vi "UHR-Fleezers Control (host) - 16.2.2v2.vi"() -> ()   [LabVIEW 2014] (continued)
                            n638 = Greater Or Equal?(x=w963, y="Dwell Duration (s)") -> (x >= y?=w970:bool)
                            n639 = local read "Dip for Protein"() -> (w967:bool)
                            n640 = Not(x=w967) -> (.not. x?=w966:bool)
                            n641 = Compound Arithmetic op=OR(w970, "Cancel dwell", w966) -> (w969:bool)
                            n642 = node-c288() -> ()  [unwired: 1 in, 1 out]
                            n643 = Select(t=FALSE, s="Pause dwell", f=w969) -> (s? t:f=w972:bool)
                            n644 = Or(x=w972, y=w964) -> (x .or. y?=w965:bool)
                            "Dwell Time (s)" <- w963
                          }
                          n645 = node-c288(w961) -> ()  [unwired: 1 out]
                        }
                      }
                    }
                  }
                }
                frame #4 {
                  n646 = local read "Dip for Protein"() -> (w982:bool)
                  n647 = local read "Dump Beads"() -> (w979:bool)
                  n648 = local write "Cancel dwell"(FALSE ("Cancel dwell")) -> ()
                  n649 = Not(x=w982) -> (.not. x?=w983:bool)
                  n650 = Not(x="Cont. Repeat Dipping?") -> (.not. x?=w985:bool)
                  n651 = Compound Arithmetic op=OR(w983, w985, w979) -> (w981:bool)
                }
              }
            }
          }
        }
      }
      event "Profile": Value Change {
        n652 = event-data() -> ()  [unwired: 1 in, 5 out]
        n653 = flat-sequence {
          tunnel: w994 -> [w997]
          tunnel: w993 -> [w1005]
          tunnel: [w999] -> w992
          tunnel: [w998] -> w991
          tunnel: [w996] -> w989
          tunnel: [w995] -> w986
          tunnel: w992 -> [w1012]
          tunnel: w991 -> [w1011]
          tunnel: [w1009] -> w990
          tunnel: w989 -> [w1010]
          tunnel: [w1008] -> w988
          tunnel: [w1007] -> w987
          tunnel: w986 -> [w1007]
          tunnel: w990 -> [w1016]
          tunnel: w988 -> [w1015]
          tunnel: w987 -> [w1014]
          frame #0 {
            n654 = call "Read Stage Position.vi"("error in"=w1005, "VISA resource name in"=w997) -> ("Current Position"=w995:cluster{dbl, dbl, dbl}, "error out"=w998:errorcluster, "VISA resource name out"=w996:refnum<visa-resource-name>)  [unwired: 1 out]
            "Current Position" <- w995
            n655 = local write "Stage Control Serial Error"(w998) -> ()
            n656 = Unbundle(w995) -> (w1002:dbl, w1004:dbl, w1000:dbl)
            n657 = Add(x=w1004, y="Y change (mm)") -> (x+y=w1001:dbl)
            n658 = Bundle(w1002, w1001, w1000) -> (w999:cluster{dbl, dbl, dbl})  [unwired: 1 in]
          }
          frame #1 {
            # "move to new position and start saving"
            n659 = local write "Stage Moving"(TRUE ("Stage Moving")) -> ()
            n660 = local write "Start Saving"(TRUE ("Start Saving")) -> ()
            n661 = call "Set Stage Position.vi"("Position"=w1012, "error in"=w1011, "VISA resource name in"=w1010) -> ("error out"=w1008:errorcluster, "VISA resource name out"=w1009:refnum<visa-resource-name>)  [unwired: 1 out]
          }
          frame #2 {
            # "go back to start"
            n662 = call "Set Stage Position.vi"("Position"=w1014, "error in"=w1015, "VISA resource name in"=w1016) -> ()  [unwired: 3 out]
          }
          frame #3 {
            # "stop saving"
            n663 = local write "Stop Saving"(TRUE ("Stop Saving")) -> ()
            n664 = local write "Stage Moving"(FALSE ("Stage Moving")) -> ()
          }
        }
      }
      event "Move to Position 1", "Move to Position 2", "Move to Position 3", "Move to Position 4", "Move to Position 5", "Lower Ch. Cap.", "Move to Position 6": Value Change {
        n665 = event-data() -> ()  [unwired: 1 in, 5 out]
        n666 = Or(x="Move to Position 5", y="Lower Ch. Cap.") -> (x .or. y?=w1023:bool)
        n667 = Build Array("Move to Position 1", "Move to Position 2", "Move to Position 3", "Move to Position 4", w1023, "Move to Position 6") -> (w1026:bool[])
        n668 = Boolean Array To Number(Boolean array=w1026) -> (number=w1025:u32)
        n669 = Logarithm Base 2(1:w1025) -> (0:w1024:dbl)
        n670 = flat-sequence {
          tunnel: w1024 -> [w1035]
          tunnel: w1021 -> [w1033]
          tunnel: w1020 -> [w1032]
          frame #0 {
            n671 = local read "Saved Stage Positions"() -> (w1043:dbl[][])
            n672 = Array Subset(array=w1043, index (row)=w1035, length (row)=1 ("length"), index (col)=1 ("index"), length (col)=3 ("length")) -> (w1040:dbl[][])
            n673 = Reshape Array(w1040, 3 ("dimension size")) -> (w1038:dbl[])
            n674 = Array To Cluster(array=w1038) -> (cluster=w1037:cluster{"[0]":dbl, "[1]":dbl, "[2]":dbl})
            n675 = call "Set Stage Position.vi"("Position"=w1037, "error in"=w1032, "VISA resource name in"=w1033) -> ("error out"=w1036:errorcluster)  [unwired: 2 out]
            n676 = local write "Stage Moving"(TRUE ("Stage Moving")) -> ()
            n677 = local write "Stage Control Serial Error"(w1036) -> ()
          }
          frame #1 {
            n678 = local write "Stage Moving"(FALSE ("Stage Moving")) -> ()
            n679 = call <vilib>:"Beep.vi"() -> ()  [unwired: 3 in, 9 out]
          }
        }
      }
      event "Got ADig bead": Value Change {
        n680 = event-data() -> ()  [unwired: 1 in, 5 out]
        n681 = flat-sequence {
          frame #0 {
            n682 = local read "Cap 1 Samp Flow ON"() -> (w1047:bool)
            n683 = case shown="True" w1047 {
              frame False {
              }
              frame True {
                n684 = property on="Sample Channel\nFlow" class="Bool (strict)"("Val(Sgnl)"=TRUE ("Value (Signaling)")) -> ()  [unwired: 2 in, 2 out]
              }
            }
          }
          frame #1 {
            n685 = property on="Inject Pump 3" class="Bool (strict)"("Val(Sgnl)"=FALSE ("Value (Signaling)")) -> ()  [unwired: 2 in, 2 out]
          }
          frame #2 {
            n686 = property on="Move Cap. 1 (DNA Bottom)" class="Bool (strict)"("Val(Sgnl)"=TRUE ("Value (Signaling)")) -> ()  [unwired: 2 in, 2 out]
          }
        }
      }
      event "Force FB Data\nScript": Value Change {
        n687 = event-data() -> ()  [unwired: 1 in, 5 out]
        n688 = flat-sequence {
          tunnel: w1056 -> [w1060]
          tunnel: w1057 -> [w1061]
          tunnel: [w1061] -> w1052
          tunnel: [w1060] -> w1051
          tunnel: w1052 -> [w1064]
          tunnel: w1051 -> [w1063]
          tunnel: ["Trap Trig Fl."] -> w1053
          tunnel: [w1089] -> w1054
          tunnel: w1053 -> [w1089]
          tunnel: [w1093] -> w1055
          tunnel: w1054 -> [w1093]
          tunnel: w1055 -> [w1095]
          frame #0 {
            n689 = property on="Trap Delta (MHz)" class="DigNum (strict)"("Val(Sgnl)"="Trap Delta Before Moving") -> ()  [unwired: 2 in, 2 out]
          }
          frame #1 {
            n690 = local read "Saved Stage Positions"() -> (w1066:dbl[][])
            n691 = property on="Trap Pos. FB Offset Factor" class="DigNum (strict)"("Val(Sgnl)"=i64 0 ("Value (Signaling)")) -> ()  [unwired: 2 in, 2 out]
            n692 = local write "FB Trap Pos Offset"(0.0 ("FB Trap Pos Offset")) -> ()
            n693 = local write "Stage Moving"(TRUE ("Stage Moving")) -> ()
            n694 = call "move to saved stage position.vi"("error in"=w1063, "Stage VISA resource name in"=w1064, "Position"="Stage Position To Establish FB", "Saved Stage Positions"=w1066) -> ("error out"=w1062:errorcluster)  [unwired: 1 out]
            n695 = local write "Stage Control Serial Error"(w1062) -> ()
          }
          frame #2 {
            n696 = call <vilib>:"Beep.vi"() -> ()  [unwired: 3 in, 9 out]
            n697 = Multiply(x="Wait (s)", y=u32 1000 ("milliseconds to wait")) -> (x*y=w1073:u32)
            n698 = property on="Trap Delta (MHz)" class="DigNum (strict)"("Val(Sgnl)"="Starting \nTrap Delta (MHz)") -> ()  [unwired: 2 in, 2 out]
            n699 = local write "Stage Moving"(FALSE ("Stage Moving")) -> ()
            n700 = Wait (ms)(milliseconds to wait=w1073) -> ()  [unwired: 1 out]
            n701 = property on="Tab Control 2" class="TabCtl (strict)"("Val(Sgnl)"=T8."Feedback on Trap Position" ("Value (Signaling)")) -> ()  [unwired: 2 in, 2 out]
            n702 = property on="Tab Control" class="TabCtl (strict)"("Val(Sgnl)"=T32."Trap Control (RF)" ("Value (Signaling)")) -> ()  [unwired: 2 in, 2 out]
          }
          frame #3 {
            n703 = property on="Set Reading to\nSetpoint" class="Bool (strict)"("Val(Sgnl)"=TRUE ("Value (Signaling)")) -> ()  [unwired: 2 in, 2 out]
            n704 = Wait (ms)(milliseconds to wait=u32 500) -> ()  [unwired: 1 out]
          }
          frame #4 {
            n705 = property on="Trap Pos. FB ON" class="Bool (strict)"("Val(Sgnl)"=TRUE ("Value (Signaling)")) -> ()  [unwired: 2 in, 2 out]
            n706 = Wait (ms)(milliseconds to wait=u32 250) -> ()  [unwired: 1 out]
          }
          frame #5 {
            n707 = case shown="False" "Trap Trig Fl." {
              frame False {
                n708 = case shown="True" "Green ON after FB ON?" {
                  selector: "Green ON after FB ON?" -> [_ w1088]
                  frame False {
                  }
                  frame True {
                    n709 = property on="Green Laser ON" class="Bool (strict)"("Val(Sgnl)"=w1088) -> ()  [unwired: 2 in, 2 out]
                  }
                }
              }
              frame True {
              }
            }
            n710 = case shown="True" "Remove Action Offset" {
              tunnel: TRUE ("Value (Signaling)") -> [w1085 w1086]
              frame False {
                n711 = property on="Remove Unwinding Offset" class="Bool (strict)"("Val(Sgnl)"=w1085) -> ()  [unwired: 2 in, 2 out]
              }
              frame True {
                n712 = property on="Remove Action Offset" class="Bool (strict)"("Val(Sgnl)"=w1086) -> ()  [unwired: 2 in, 2 out]
              }
            }
            n713 = Wait (ms)(milliseconds to wait=u32 250) -> ()  [unwired: 1 out]
          }
          frame #6 {
            n714 = property on="Start Saving" class="Bool (strict)"("Val(Sgnl)"=TRUE ("Value (Signaling)")) -> ()  [unwired: 2 in, 2 out]
            n715 = Wait (ms)(milliseconds to wait=u32 5000) -> ()  [unwired: 1 out]
          }
          frame #7 {
            w1092 = TRUE ("Value (Signaling)")
            n716 = property on="Rem fb disp offset" class="Bool (strict)"("Val(Sgnl)"=w1092) -> ()  [unwired: 2 in, 2 out]
            n717 = property on="Remove Offset" class="Bool (strict)"("Val(Sgnl)"=w1092) -> ()  [unwired: 2 in, 2 out]
            n718 = Wait (ms)(milliseconds to wait=u32 100) -> ()  [unwired: 1 out]
          }
          frame #8 {
            n719 = case shown="True" w1095 {
              frame False {
              }
              frame True {
                n720 = local write "Trap Trig. Fl."(TRUE ("Value (Signaling)")) -> ()
              }
            }
          }
          frame #9 {
            n721 = case shown="True" "Start dipping after?" {
              frame False {
              }
              frame True {
                n722 = flat-sequence {
                  frame #0 {
                    n723 = Multiply(x="Delay before dipping (s)", y=1000.0) -> (x*y=w1099:dbl)
                    n724 = Wait (ms)(milliseconds to wait=w1099) -> ()  [unwired: 1 out]
                  }
                  frame #1 {
                    n725 = property on="Dip for Protein" class="Bool (strict)"("Val(Sgnl)"=TRUE ("Value (Signaling)")) -> ()  [unwired: 2 in, 2 out]
                    n726 = local write "Scripts"(T33."Dipping" ("Scripts")) -> ()
                  }
                }
              }
            }
          }
        }
      }
      event "Start lifetime measurements": Value Change {
        n727 = event-data() -> ()  [unwired: 1 in, 5 out]
        n728 = local write "Start lifetime measurements"(FALSE ("Start lifetime measurements")) -> ()
        n729 = flat-sequence {
          tunnel: w1104 -> [w1107]
          tunnel: [w1107] -> w1103
          tunnel: w1103 -> [w1114]
          frame #0 {
            # "This will:\n1) stop reading trap pos fifo\n2) start sending zeros to trap position host data\nWait a second because may be in the middle of\nwaiting for FIFO data."
            n730 = local write "Trap positions to FIFO"(FALSE ("Trap positions to FIFO")) -> ()
            n731 = Wait (ms)(milliseconds to wait=u32 1000) -> ()  [unwired: 1 out]
          }
          frame #1 {
            w1113 = FALSE ("Trap Pos to FIFO")
            # "Send lifetimes to FIFO"
            # "Stop and restart FIFO to clear"
            # "On FPGA, stop sending trap\nposition data to FIFO and make\nsure lifetimes aren't sent to FIFO\neither"
            n732 = xnode "Read/Write Control"("FPGA VI Reference In"=w1114, "Trap Pos to FIFO"=w1113, "Lifetime to FIFO"=w1113, "lifetime events in fifo"=u16 0) -> ("FPGA VI Reference Out"=w1115:T25)  [unwired: 1 in, 1 out]
            n733 = xnode "Invoke Method"("FPGA VI Reference In"=w1115) -> ("FPGA VI Reference Out"=w1112:T25)  [unwired: 1 in, 1 out]
            n734 = xnode "Invoke Method"("FPGA VI Reference In"=w1112) -> ("FPGA VI Reference Out"=w1111:T25)  [unwired: 1 in, 1 out]
            n735 = xnode "Read/Write Control"("FPGA VI Reference In"=w1111, "Lifetime to FIFO"=TRUE) -> ()  [unwired: 1 in, 2 out]
          }
          frame #2 {
            "Measuring lifetimes" <- TRUE ("Measuring lifetimes")
          }
        }
      }
      event "Stop lifetime measurements": Value Change {
        n736 = event-data() -> ()  [unwired: 1 in, 5 out]
        n737 = local write "Stop lifetime measurements"(FALSE ("Stop lifetime measurements")) -> ()
        n738 = flat-sequence {
          tunnel: w1117 -> [w1126]
          frame #0 {
            n739 = local write "Measuring lifetimes"(FALSE ("Measuring lifetimes")) -> ()
          }
          frame #1 {
            # "clear fifo count"
            # "Start sending trap position\ndata to FIFO"
            # "Stop sending lifetime data\nto FIFO"
            n740 = xnode "Read/Write Control"("FPGA VI Reference In"=w1126, "Lifetime to FIFO"=FALSE ("Trap Pos to FIFO")) -> ("FPGA VI Reference Out"=w1125:T25)  [unwired: 1 in, 1 out]
            n741 = xnode "Read/Write Control"("FPGA VI Reference In"=w1125, "Trap Pos to FIFO"=TRUE) -> ("FPGA VI Reference Out"=w1122:T25, "lifetime events in fifo"=w1123:u16)  [unwired: 1 in, 1 out]
            n742 = xnode "Read/Write Control"("FPGA VI Reference In"=w1122, "Lifetime events to read blue"=w1123) -> ("FPGA VI Reference Out"=w1121:T25)  [unwired: 1 in, 1 out]
            n743 = xnode "Read/Write Control"("FPGA VI Reference In"=w1121, "Lifetime read blue fifo"=TRUE) -> ()  [unwired: 1 in, 2 out]
          }
          frame #2 {
            # "Reset data stream (clears all FIFO's\nand resynchronizes)\nWait a second to make sure everything\nis running before switching to real data"
            n744 = local write "Reset"(TRUE ("Reset")) -> ()
            n745 = Wait (ms)(milliseconds to wait=u32 1000) -> ()  [unwired: 1 out]
          }
          frame #3 {
            n746 = local write "Trap positions to FIFO"(TRUE ("Trap positions to FIFO")) -> ()
            n747 = Wait (ms)(milliseconds to wait=u32 1000) -> ()  [unwired: 1 out]
          }
          frame #4 {
            # "Need a second reset\nfor some reason (not\nclear why)"
            n748 = local write "Reset"(TRUE ("Reset")) -> ()
          }
        }
      }
      event "Fixed Traps Data\nScript": Value Change {
        n749 = event-data() -> ()  [unwired: 1 in, 5 out]
        n750 = flat-sequence {
          frame #0 {
            n751 = case shown="True" "Green ON" {
              frame False {
              }
              frame True {
                n752 = property on="Green Laser ON" class="Bool (strict)"("Val(Sgnl)"=TRUE) -> ()  [unwired: 2 in, 2 out]
              }
            }
            n753 = local write "Offset (nm)"(0.0 ("Offset (nm)")) -> ()
            n754 = property on="Sample Channel\nFlow" class="Bool (strict)"("Val(Sgnl)"=FALSE ("Value (Signaling)")) -> ()  [unwired: 2 in, 2 out]
            n755 = property on="Trap Delta (MHz)" class="DigNum (strict)"("Val(Sgnl)"="Fixed Traps Trap Delta (MHz)") -> ()  [unwired: 2 in, 2 out]
          }
          frame #1 {
            n756 = Wait (ms)(milliseconds to wait=u32 1000) -> ()  [unwired: 1 out]
          }
          frame #2 {
            n757 = local write "Start Saving"(TRUE ("Start Saving")) -> ()
          }
          frame #3 {
            n758 = local read "Bead Sep. Int. Time (s)"() -> (w1140:dbl)
            n759 = Multiply(x=w1140, y=1000.0) -> (x*y=w1142:dbl)
            n760 = Wait (ms)(milliseconds to wait=w1142) -> ()  [unwired: 1 out]
          }
          frame #4 {
            n761 = property on="Remove Offset" class="Bool (strict)"("Val(Sgnl)"=TRUE ("Value (Signaling)")) -> ()  [unwired: 2 in, 2 out]
          }
          frame #5 {
            n762 = property on="Dip for Protein" class="Bool (strict)"("Val(Sgnl)"="Start dipping after?") -> ()  [unwired: 2 in, 2 out]
          }
        }
      }
      event "Got DNA bead": Value Change {
        n763 = event-data() -> ()  [unwired: 1 in, 5 out]
        n764 = flat-sequence {
          frame #0 {
            n765 = local read "Daq spot flow on"() -> (w1147:bool)
            n766 = case shown="True" w1147 {
              frame False {
              }
              frame True {
                n767 = property on="Sample Channel\nFlow" class="Bool (strict)"("Val(Sgnl)"=TRUE ("Value (Signaling)")) -> ()  [unwired: 2 in, 2 out]
              }
            }
            n768 = property on="Got DNA bead" class="Bool"("Key Focus"=FALSE) -> ()  [unwired: 2 in, 2 out]
          }
          frame #1 {
            n769 = property on="Inject Pump 1" class="Bool (strict)"("Val(Sgnl)"=FALSE ("Value (Signaling)")) -> ()  [unwired: 2 in, 2 out]
          }
          frame #2 {
            n770 = property on="Cal/Data Acq. Spot" class="Bool (strict)"("Val(Sgnl)"=TRUE ("Value (Signaling)")) -> ()  [unwired: 2 in, 2 out]
          }
        }
      }
      event "Take Stepping Data": Value Change {
        n771 = event-data() -> ()  [unwired: 1 in, 5 out]
        n772 = local read "Save ave N"() -> (w1159:dbl)
        n773 = flat-sequence {
          tunnel: w1159 -> [w1161]
          tunnel: [w1161] -> w1154
          tunnel: [w1163] -> w1155
          tunnel: w1154 -> [w1163]
          tunnel: [w1165] -> w1156
          tunnel: w1155 -> [w1165]
          tunnel: [w1168] -> w1157
          tunnel: w1156 -> [w1168]
          tunnel: [w1170] -> w1158
          tunnel: w1157 -> [w1170]
          tunnel: [w1172] -> w1152
          tunnel: w1158 -> [w1172]
          tunnel: w1152 -> [w1175]
          tunnel: [w1175] -> w1151
          tunnel: w1151 -> [w1176]
          tunnel: [w1176] -> w1153
          tunnel: w1153 -> [w1182]
          frame #0 {
            n774 = property on="Save ave N" class="DigNum (strict)"("Val(Sgnl)"="Save ave factor") -> ()  [unwired: 2 in, 2 out]
          }
          frame #1 {
            n775 = Wait (ms)(milliseconds to wait=u32 100) -> ()  [unwired: 1 out]
          }
          frame #2 {
            n776 = local read "Offset 2 Start (MHz)"() -> (w1167:dbl)
            n777 = property on="Saved AOD Raster Scan Parameter Sets" class="Arr (strict)"("Index Values"=u32[] [2]) -> ()  [unwired: 2 in, 2 out]
            n778 = property on="Trap Delta (MHz)" class="DigNum (strict)"("Val(Sgnl)"=w1167) -> ()  [unwired: 2 in, 2 out]
          }
          frame #3 {
            n779 = property on="Load parameters" class="Bool (strict)"("Val(Sgnl)"=TRUE ("Value (Signaling)")) -> ()  [unwired: 2 in, 2 out]
          }
          frame #4 {
            n780 = Wait (ms)(milliseconds to wait=u32 100) -> ()  [unwired: 1 out]
          }
          frame #5 {
            n781 = property on="Trap Raster Scan" class="Bool (strict)"("Val(Sgnl)"=TRUE ("Value (Signaling)")) -> ()  [unwired: 2 in, 2 out]
          }
          frame #6 {
            n782 = Wait (ms)(milliseconds to wait=u32 1000) -> ()  [unwired: 1 out]
          }
          frame #7 {
            n783 = while {
              stop <- w1179 stop-if-true
              n784 = local read "Raster Scanning..."() -> (w1181:bool)
              n785 = local read "Saving..."() -> (w1180:bool)
              n786 = Not(x=w1180) -> (.not. x?=w1177:bool)
              n787 = Not(x=w1181) -> (.not. x?=w1178:bool)
              n788 = And(x=w1178, y=w1177) -> (x .and. y?=w1179:bool)
            }
          }
          frame #8 {
            n789 = property on="Save ave N" class="DigNum (strict)"("Val(Sgnl)"=w1182) -> ()  [unwired: 2 in, 2 out]
          }
        }
      }
      event "Step Size (nm)": Value Change {
        n790 = event-data() -> ()  [unwired: 1 in, 5 out]
        n791 = flat-sequence {
          frame #0 {
            n792 = property on="Saved AOD Raster Scan Parameter Sets" class="Arr (strict)"("Index Values"=u32[] [1]) -> ()  [unwired: 2 in, 2 out]
          }
          frame #1 {
            n793 = Multiply(x="N Steps", y="Step Size (nm)") -> (x*y=w1184:dbl)
            n794 = property on="Scan Speed AOD (nm/s) 2" class="DigNum (strict)"("Value"="Step Size (nm)") -> ()  [unwired: 2 in, 2 out]
            n795 = property on="Step Size AOD (nm) 2" class="DigNum (strict)"("Value"="Step Size (nm)") -> ()  [unwired: 2 in, 2 out]
            n796 = property on="Scan Range AOD (nm) 2" class="DigNum (strict)"("Value"=w1184) -> ()  [unwired: 2 in, 2 out]
          }
        }
      }
      event "Take Detection Laser\nImage": Value Change {
        n797 = event-data() -> ()  [unwired: 1 in, 5 out]
        n798 = local read "RF BD 2 to green AOM"() -> (w1214:bool)
        n799 = flat-sequence {
          tunnel: [w1245] -> w1231
          tunnel: [w1244] -> w1224
          tunnel: [w1243] -> w1216
          tunnel: [w1242] -> w1215
          tunnel: w1214 -> [w1242]
          tunnel: [w1241] -> w1201
          tunnel: [w1240] -> w1194
          tunnel: [w1239] -> w1187
          tunnel: [w1252] -> w1232
          tunnel: w1231 -> [w1252]
          tunnel: [w1251] -> w1225
          tunnel: w1224 -> [w1251]
          tunnel: [w1250] -> w1217
          tunnel: w1216 -> [w1250]
          tunnel: w1215 -> [w1249]
          tunnel: [w1249] -> w1213
          tunnel: [w1248] -> w1202
          tunnel: w1201 -> [w1248]
          tunnel: [w1247] -> w1195
          tunnel: w1194 -> [w1247]
          tunnel: [w1246] -> w1188
          tunnel: w1187 -> [w1246]
          tunnel: [w1260] -> w1233
          tunnel: w1232 -> [w1260]
          tunnel: [w1259] -> w1226
          tunnel: w1225 -> [w1259]
          tunnel: [w1258] -> w1218
          tunnel: w1217 -> [w1258]
          tunnel: w1213 -> [w1257]
          tunnel: [w1257] -> w1208
          tunnel: [w1256] -> w1203
          tunnel: w1202 -> [w1256]
          tunnel: [w1255] -> w1196
          tunnel: w1195 -> [w1255]
          tunnel: [w1254] -> w1189
          tunnel: w1188 -> [w1254]
          tunnel: [w1271] -> w1234
          tunnel: w1233 -> [w1271]
          tunnel: [w1270] -> w1227
          tunnel: w1226 -> [w1270]
          tunnel: [w1269] -> w1219
          tunnel: w1218 -> [w1269]
          tunnel: [w1268] -> w1209
          tunnel: w1208 -> [w1268]
          tunnel: [w1267] -> w1204
          tunnel: w1203 -> [w1267]
          tunnel: [w1266] -> w1197
          tunnel: w1196 -> [w1266]
          tunnel: [w1265] -> w1190
          tunnel: w1189 -> [w1265]
          tunnel: [w1279] -> w1235
          tunnel: w1234 -> [w1279]
          tunnel: [w1278] -> w1228
          tunnel: w1227 -> [w1278]
          tunnel: [w1277] -> w1220
          tunnel: w1219 -> [w1277]
          tunnel: [w1276] -> w1210
          tunnel: w1209 -> [w1276]
          tunnel: [w1275] -> w1205
          tunnel: w1204 -> [w1275]
          tunnel: [w1274] -> w1198
          tunnel: w1197 -> [w1274]
          tunnel: [w1273] -> w1191
          tunnel: w1190 -> [w1273]
          tunnel: [w1287] -> w1236
          tunnel: w1235 -> [w1287]
          tunnel: [w1286] -> w1229
          tunnel: w1228 -> [w1286]
          tunnel: [w1285] -> w1221
          tunnel: w1220 -> [w1285]
          tunnel: [w1284] -> w1211
          tunnel: w1210 -> [w1284]
          tunnel: [w1283] -> w1206
          tunnel: w1205 -> [w1283]
          tunnel: [w1282] -> w1199
          tunnel: w1198 -> [w1282]
          tunnel: [w1281] -> w1192
          tunnel: w1191 -> [w1281]
          tunnel: [w1295] -> w1237
          tunnel: w1236 -> [w1295]
          tunnel: [w1294] -> w1230
          tunnel: w1229 -> [w1294]
          tunnel: [w1293] -> w1222
          tunnel: w1221 -> [w1293]
          tunnel: [w1292] -> w1212
          tunnel: w1211 -> [w1292]
          tunnel: [w1291] -> w1207
          tunnel: w1206 -> [w1291]
          tunnel: [w1290] -> w1200
          tunnel: w1199 -> [w1290]
          tunnel: [w1289] -> w1193
          tunnel: w1192 -> [w1289]
          tunnel: w1237 -> [w1305]
          tunnel: w1230 -> [w1304]
          tunnel: [w1302] -> w1223
          tunnel: w1222 -> [w1302]
          tunnel: w1212 -> [w1301]
          tunnel: w1207 -> [w1300]
          tunnel: w1200 -> [w1299]
          tunnel: w1193 -> [w1298]
          tunnel: w1223 -> [w1309]
          frame #0 {
            # "when RF synth controls green AOM"
            n800 = local read "Laser interlacing mode"() -> (w1244:enum32{"Laser ON", "Laser OFF", "Interlace"})
            n801 = local read "BD 2 Amplitude 1 (%)"() -> (w1241:dbl)
            n802 = local read "BD 2 Amplitude 2 (%)"() -> (w1240:dbl)
            n803 = local read "BD 2 Amplitude 3 (%)"() -> (w1239:dbl)
            n804 = local read "Green FB On/Off"() -> (w1243:bool)
            n805 = local read "Green Laser ON"() -> (w1245:bool)
          }
          frame #1 {
            n806 = property on="Green FB On/Off" class="Bool (strict)"("Val(Sgnl)"=FALSE ("Value (Signaling)")) -> ()  [unwired: 2 in, 2 out]
          }
          frame #2 {
            n807 = case "RF synth BD controls green AOM" shown="True" w1257 {
              frame False {
              }
              frame True {
                w1264 = 30.0 ("Value (Signaling)")
                n808 = property on="BD 2 Amplitude 2 (%)" class="DigNum (strict)"("Val(Sgnl)"=w1264) -> ()  [unwired: 2 in, 2 out]
                n809 = property on="BD 2 Amplitude 1 (%)" class="DigNum (strict)"("Val(Sgnl)"=w1264) -> ()  [unwired: 2 in, 2 out]
                n810 = property on="BD 2 Amplitude 3 (%)" class="DigNum (strict)"("Val(Sgnl)"=w1264) -> ()  [unwired: 2 in, 2 out]
              }
            }
            n811 = property on="Green Laser ON" class="Bool (strict)"("Val(Sgnl)"=TRUE ("Value (Signaling)")) -> ()  [unwired: 2 in, 2 out]
            n812 = property on="Flip Green Filter" class="Bool (strict)"("Val(Sgnl)"=TRUE ("Value (Signaling)")) -> ()  [unwired: 2 in, 2 out]
            n813 = property on="Laser interlacing mode" class="RadioBtnsControl (strict)"("Val(Sgnl)"=enum32{"Laser ON", "Laser OFF", "Interlace"}."Laser ON" ("Value (Signaling)")) -> ()  [unwired: 2 in, 2 out]
          }
          frame #3 {
            n814 = Wait (ms)(milliseconds to wait=u32 500) -> ()  [unwired: 1 out]
          }
          frame #4 {
            n815 = property on="Confocal Image" class="Bool (strict)"("Val(Sgnl)"=TRUE ("Value (Signaling)")) -> ()  [unwired: 2 in, 2 out]
          }
          frame #5 {
            n816 = Wait (ms)(milliseconds to wait=u32 2000) -> ()  [unwired: 1 out]
          }
          frame #6 {
            n817 = while {
              stop <- w1296 stop-if-true
              n818 = local read "Saving..."() -> (w1297:bool)
              n819 = Not(x=w1297) -> (.not. x?=w1296:bool)
            }
          }
          frame #7 {
            n820 = case shown="True" w1301 {
              tunnel: w1300 -> [_ w1308]
              tunnel: w1299 -> [_ w1307]
              tunnel: w1298 -> [_ w1306]
              frame False {
              }
              frame True {
                n821 = property on="BD 2 Amplitude 1 (%)" class="DigNum (strict)"("Val(Sgnl)"=w1308) -> ()  [unwired: 2 in, 2 out]
                n822 = property on="BD 2 Amplitude 2 (%)" class="DigNum (strict)"("Val(Sgnl)"=w1307) -> ()  [unwired: 2 in, 2 out]
                n823 = property on="BD 2 Amplitude 3 (%)" class="DigNum (strict)"("Val(Sgnl)"=w1306) -> ()  [unwired: 2 in, 2 out]
              }
            }
            n824 = property on="Green Laser ON" class="Bool (strict)"("Val(Sgnl)"=w1305) -> ()  [unwired: 2 in, 2 out]
            n825 = property on="Flip Green Filter" class="Bool (strict)"("Val(Sgnl)"=TRUE ("Value (Signaling)")) -> ()  [unwired: 2 in, 2 out]
            n826 = property on="Laser interlacing mode" class="RadioBtnsControl (strict)"("Val(Sgnl)"=w1304) -> ()  [unwired: 2 in, 2 out]
          }
          frame #8 {
            n827 = property on="Green FB On/Off" class="Bool (strict)"("Val(Sgnl)"=w1309) -> ()  [unwired: 2 in, 2 out]
          }
        }
      }
      event "Move in a Circle": Value Change {
        w1311 = dbl[] []
        # "converting distance (d) to angle (a)\na=arcsin(d/2r)"
        # "radius"
        # "radius"
        # "T1 Y"
        # "T1 X"
        n828 = event-data() -> ()  [unwired: 1 in, 5 out]
        n829 = local read "BD 1 Frequency 1 (MHz)"() -> (w1319:dbl)
        n830 = local read "BD 2 Frequency 1 (MHz)"() -> (w1318:dbl)
        n831 = local read "BD 1 Frequency 2 (MHz)"() -> (w1317:dbl)
        n832 = local read "BD 2 Frequency 2 (MHz)"() -> (w1316:dbl)
        n833 = Subtract(x=w1318, y="Center Y Frequency (MHz)") -> (x-y=w1323:dbl)
        n834 = Absolute Value(x=w1323) -> (abs(x)=w1314:dbl)
        n835 = flat-sequence {
          tunnel: w1314 -> [w1326]
          tunnel: [w1326] -> w1313
          frame #0 {
            n836 = local write "Radius (MHz)"(w1326) -> ()
          }
        }
        n837 = node-c288("Time step (ms)") -> (w1325:T28)  [unwired: 3 in]
        n838 = timed-loop {
          timing: w1325 -> [_]
          timing-out: [_] -> w1324
          tunnel: w1319 -> [w1417]
          tunnel: w1318 -> [_]
          tunnel: w1317 -> [w1421]
          tunnel: w1316 -> [_]
          tunnel: "Center Y Frequency (MHz)" -> [w1410]
          shift-right: [w1371] -> _
          shift-left: w1311 -> [w1378]
          shift-right: [w1369] -> _
          shift-left: w1311 -> [w1377]
          shift-right: [w1362] -> _
          shift-left: w1311 -> [w1375]
          shift-right: [w1360] -> _
          shift-left: w1311 -> [w1374]
          tunnel: "Move in a Circle" -> [_]
          tunnel: ["Back to start on finish?"] -> w1315
          tunnel: w1313 -> [_]
          tunnel: w1312 -> [w1392]
          tunnel: w1311 -> [w1373]
          shift-right: [w1344] -> _
          shift-left: 0.0 -> [w1342]
          i -> [w1351]
          stop <- w1415 stop-if-true
          w1359 = 0 ("index")
          w1380 = 1 ("dimension size")
          # "Keep phase within\n2pi so errors don't \nbuild"
          # "Accumulated\nphase"
          # "Current phase"
          # "Trap 2"
          # "Trap 1"
          # "ignore if N = 0"
          # "r"
          # "r"
          # "r"
          # "r"
          # "\"omega*t\""
          # "Trap 2"
          # "Trap separation (radians)"
          # "Trap 1"
          # "Offset (starts\n at bottom of\n the circle)"
          # "omega"
          n839 = node-c288() -> (w1428:i64)  [unwired: 1 in]
          n840 = Divide(x=w1428, y=1000) -> (x/y=w1347:dbl)
          n841 = Divide(x="2D Motion Trap Separation (MHz)", y="Radius (MHz)") -> (x/y=w1402:dbl)
          n842 = Negate(x=w1347) -> (-x=w1346:dbl)
          n843 = Divide(x="Trap 2 phase shift (deg)", y=360.0) -> (x/y=w1393:dbl)
          n844 = Inverse Sine(1:w1402) -> (0:w1338:dbl)
          n845 = Multiply(x=6.283185307179586, y=w1393) -> (x*y=w1339:dbl)
          n846 = Multiply(x=6.283185307179586, y="2D Motion Frequency (Hz)") -> (x*y=w1350:dbl)
          n847 = Select(t=w1347, s="Counterclockwise/Clockwise", f=w1346) -> (s? t:f=w1349:dbl)
          n848 = Multiply(x=w1350, y=w1349) -> (x*y=w1340:dbl)
          n849 = Select(t=w1338, s="Trap shift\nmethod", f=w1339) -> (s? t:f=w1337:dbl)
          n850 = Add(x=w1340, y=w1342) -> (x+y=w1343:dbl)
          n851 = Add(x=w1343, y=w1337) -> (x+y=w1399:dbl)
          n852 = Add(x=w1343, y=1.5707963267948966) -> (x+y=w1348:dbl)
          n853 = Add(x=w1399, y=1.5707963267948966) -> (x+y=w1412:dbl)
          n854 = Cosine(x=w1348) -> (cos(x)=w1426:dbl)
          n855 = Sine(x=w1348) -> (sin(x)=w1425:dbl)
          n856 = Multiply(x=w1426, y="Radius (MHz)") -> (x*y=w1419:dbl)
          n857 = Cosine(x=w1412) -> (cos(x)=w1424:dbl)
          n858 = Sine(x=w1412) -> (sin(x)=w1423:dbl)
          n859 = Multiply(x=w1425, y="Radius (MHz)") -> (x*y=w1418:dbl)
          n860 = Multiply(x=w1424, y="Radius (MHz)") -> (x*y=w1422:dbl)
          n861 = Multiply(x=w1423, y="Radius (MHz)") -> (x*y=w1420:dbl)
          n862 = Add(x=w1419, y=w1417) -> (x+y=w1368:dbl)
          n863 = Add(x=w1418, y=w1410) -> (x+y=w1366:dbl)
          n864 = Greater Or Equal?(x=w1351, y="N steps then stop") -> (x >= y?=w1409:bool)
          n865 = Add(x=w1422, y=w1421) -> (x+y=w1357:dbl)
          n866 = Add(x=w1420, y=w1410) -> (x+y=w1355:dbl)
          n867 = Not Equal To 0?(x="N steps then stop") -> (x != 0?=w1405:bool)
          n868 = And(x=w1409, y=w1405) -> (x .and. y?=w1406:bool)
          n869 = local read "Trap 1 sum mean"() -> (w1389:dbl)
          n870 = local read "Stop All"() -> (w1414:bool)
          n871 = local write "BD 1 Frequency 1 (MHz)"(w1368) -> ()
          n872 = local write "BD 2 Frequency 1 (MHz)"(w1366) -> ()
          n873 = local write "BD 1 Frequency 2 (MHz)"(w1357) -> ()
          n874 = local write "BD 2 Frequency 2 (MHz)"(w1355) -> ()
          n875 = Select(t=w1351, s="test", f=w1389) -> (s? t:f=→"Waveform Chart":dbl)
          n876 = Compound Arithmetic op=OR(w1414, "Stop Moving", w1406) -> (w1415:bool)
          n877 = local read "BD 1 Frequency 3 (MHz)"() -> (w1398:dbl)
          n878 = local read "BD 2 Frequency 3 (MHz)"() -> (w1397:dbl)
          n879 = Select(t=w1373, s="Reset graph", f=w1374) -> (s? t:f=w1354:dbl[])
          n880 = Select(t=w1373, s="Reset graph", f=w1375) -> (s? t:f=w1356:dbl[])
          n881 = Select(t=w1373, s="Reset graph", f=w1377) -> (s? t:f=w1365:dbl[])
          n882 = Select(t=w1373, s="Reset graph", f=w1378) -> (s? t:f=w1367:dbl[])
          n883 = Initialize Array(w1355, w1380) -> (w1381:dbl[])
          n884 = Initialize Array(w1366, w1380) -> (w1384:dbl[])
          n885 = Initialize Array(w1357, w1380) -> (w1382:dbl[])
          n886 = Initialize Array(w1368, w1380) -> (w1385:dbl[])
          n887 = local read "Y RF Frequency Limits (MHz)"() -> (w1395:T18)
          n888 = local read "X RF Frequency Limits (MHz)"() -> (w1396:T18)
          n889 = call "set RF board frequency - interlace.vi"("Board 2 Frequency Limits"=w1395, "Board 1 Frequency Limits"=w1396, "FPGA VI Reference In"=w1392, "Board 2 Frequency 3 (MHz)"=w1397, "Board 1 Frequency 3 (MHz)"=w1398, "Board 2 Frequency 2 (MHz)"=w1355, "Board 2 Frequency 1 (MHz)"=w1366, "Board 1 Frequency 2 (MHz)"=w1357, "Board 1 Frequency 1  (MHz)"=w1368) -> ()  [unwired: 1 in, 2 out]
          n890 = Bundle(w1382, w1381) -> (w1353:cluster{dbl[], dbl[]})  [unwired: 1 in]
          n891 = Bundle(w1385, w1384) -> (w1383:cluster{dbl[], dbl[]})  [unwired: 1 in]
          n892 = Build Array (concatenate)(w1368, w1367) -> (w1372:dbl[])
          n893 = Build Array (concatenate)(w1366, w1365) -> (w1370:dbl[])
          n894 = Build Array (concatenate)(w1357, w1356) -> (w1363:dbl[])
          n895 = Build Array (concatenate)(w1355, w1354) -> (w1361:dbl[])
          n896 = Bundle(w1372, w1370) -> (w1352:cluster{dbl[], dbl[]})  [unwired: 1 in]
          n897 = Bundle(w1363, w1361) -> (w1379:cluster{dbl[], dbl[]})  [unwired: 1 in]
          n898 = Build Array(w1383, w1353, w1352, w1379) -> (→"Trap trajectories":cluster{dbl[], dbl[]}[])
          n899 = case "To pause the process" shown="True" "Pause rotation" {
            frame False {
            }
            frame True {
              n900 = while {
                stop <- w1431 stop-if-true
                n901 = local read "Pause rotation"() -> (w1432:bool)
                n902 = Wait (ms)(milliseconds to wait=u32 10) -> ()  [unwired: 1 out]
                n903 = Not(x=w1432) -> (.not. x?=w1431:bool)
              }
            }
          }
          n904 = Decrement(x="N steps to plot") -> (x-1=w1358:i32)
          n905 = Array Subset(array=w1370, index=w1359, length=w1358) -> (w1369:dbl[])
          n906 = Array Subset(array=w1372, index=w1359, length=w1358) -> (w1371:dbl[])
          n907 = Array Subset(array=w1363, index=w1359, length=w1358) -> (w1362:dbl[])
          n908 = Array Subset(array=w1361, index=w1359, length=w1358) -> (w1360:dbl[])
          n909 = Quotient & Remainder(x=w1343, y=6.283185307179586) -> (x-y*floor(x/y)=w1344:dbl)  [unwired: 1 out]
          n910 = node-c288() -> ()  [unwired: 1 in, 1 out]
        }
        n911 = node-c288(w1324) -> ()  [unwired: 1 out]
        n912 = case shown="True" w1315 {
          tunnel: w1319 -> [_ w1330]
          tunnel: w1318 -> [_ w1329]
          tunnel: w1317 -> [_ w1328]
          tunnel: w1316 -> [_ w1327]
          frame False {
          }
          frame True {
            n913 = flat-sequence {
              tunnel: w1330 -> [w1334]
              tunnel: w1329 -> [w1333]
              tunnel: w1328 -> [w1332]
              tunnel: w1327 -> [w1331]
              frame #0 {
                n914 = local write "BD 1 Frequency 1 (MHz)"(w1334) -> ()
                n915 = local write "BD 2 Frequency 1 (MHz)"(w1333) -> ()
                n916 = local write "BD 1 Frequency 2 (MHz)"(w1332) -> ()
                n917 = local write "BD 2 Frequency 2 (MHz)"(w1331) -> ()
              }
              frame #1 {
                n918 = property on="Update all trap values" class="Bool (strict)"("Val(Sgnl)"=TRUE ("Value (Signaling)")) -> ()  [unwired: 2 in, 2 out]
              }
            }
          }
        }
      }
      event "Stop All": Value Change {
        # "Stopping blue laser before shutting off program"
        n919 = event-data() -> ()  [unwired: 1 in, 5 out]
        n920 = local read "Delay (ms)"() -> (w1442:i32)
        n921 = call "serial write macro.vi"("String"="l0", "Delay (ms)"=w1442, "VISA resource name"=w1445) -> ("read buffer"=w1440:string, "error out"=w1441:errorcluster, "VISA resource name out"=w1444:refnum<visa-resource-name>)
        n922 = local write "read blue buffer"(w1440) -> ()
        n923 = local write "Blue Error Out"(w1441) -> ()
        n924 = VISA Close(VISA resource name=w1444) -> ()  [unwired: 1 in, 1 out]
        n925 = local read "Stop All"() -> (w1446:bool)
      }
      event "Sensitivity", "Offset Current Sign", "Offset Current Value", "Offset Current", "Bias Voltage", "Bias Voltage (mV)", "Filter Type", "Lowpass 3dB Point", "Highpass 3dB Point", "Filter Reset", "Invert Signal", "Gain Mode", "Send Command": Value Change {
        w1453 = 250 ("Delay (ms)")
        n926 = event-data() -> ()  [unwired: 1 in, 5 out]
        n927 = event shown="[0] \"Sensitivity\": Value Change" {
          selector: _ -> [_ _ _ _ _ _ _ _ _ _ _ _ _]
          dyn-events: _ -> [_ _ _ _ _ _ _ _ _ _ _ _ _]
          timeout: _ -> [_ _ _ _ _ _ _ _ _ _ _ _ _]
          tunnel: [w1465 w1473 w1481 w1490 w1500 w1508 w1511 w1515 w1518 w1521 w1524 w1531 "Command"] -> w1452
          tunnel: [w1460 w1467 w1477 w1484 w1494 w1504 _ _ _ _ _ w1527 _] -> w1447
          event "Sensitivity": Value Change {
            n928 = event-data() -> ()  [unwired: 1 in, 5 out]
            n929 = property on="Sensitivity" class="CmbBox"() -> ("Value"=→"Gain":string)  [unwired: 2 in, 2 out]
            n930 = Concatenate Strings("SENS ", "Sensitivity") -> (w1465:string)
            n931 = local read "Gain"() -> (w1462:string)
            n932 = Concatenate Strings("gain set at ", w1462) -> (w1460:string)
          }
          event "Offset Current Sign": Value Change {
            n933 = event-data() -> ()  [unwired: 1 in, 4 out]
            n934 = Boolean To (0,1)(Boolean="Offset Current Sign") -> (0, 1=w1476:i16)
            n935 = Select(t="positive", s="Offset Current Sign", f="negative") -> (s? t:f=w1468:string)
            n936 = Number To Decimal String(number=w1476) -> (decimal integer string=w1475:string)  [unwired: 1 in]
            n937 = Concatenate Strings("IOSN " ("string"), w1475) -> (w1473:string)
            n938 = Concatenate Strings("offset current sign ", w1468) -> (w1467:string)
          }
          event "Offset Current Value": Value Change {
            n939 = event-data() -> ()  [unwired: 1 in, 5 out]
            n940 = property on="Offset Current Value" class="CmbBox"() -> ("Value"=→"Read offset current":string)  [unwired: 2 in, 2 out]
            n941 = local read "Read offset current"() -> (w1478:string)
            n942 = Concatenate Strings("IOLV ", "Offset Current Value") -> (w1481:string)
            n943 = Concatenate Strings("offset current value ", w1478) -> (w1477:string)
          }
          event "Offset Current": Value Change {
            n944 = event-data() -> ()  [unwired: 1 in, 5 out]
            n945 = Boolean To (0,1)(Boolean="Offset Current") -> (0, 1=w1493:i16)
            n946 = Select(t="on", s="Offset Current", f="off") -> (s? t:f=w1485:string)
            n947 = Number To Decimal String(number=w1493) -> (decimal integer string=w1492:string)  [unwired: 1 in]
            n948 = Concatenate Strings("IOON " ("string"), w1492) -> (w1490:string)
            n949 = Concatenate Strings("offset current ", w1485) -> (w1484:string)
          }
          event "Bias Voltage": Value Change {
            n950 = event-data() -> ()  [unwired: 1 in, 5 out]
            n951 = Boolean To (0,1)(Boolean="Bias Voltage") -> (0, 1=w1501:i16)
            n952 = Number To Decimal String(number=w1501) -> (decimal integer string=w1502:string)  [unwired: 1 in]
            n953 = Select(t="on", s="Bias Voltage", f="off") -> (s? t:f=w1495:string)
            n954 = Concatenate Strings("BSON " ("string"), w1502) -> (w1500:string)
            n955 = Concatenate Strings("bias voltage", w1495) -> (w1494:string)
          }
          event "Bias Voltage (mV)": Value Change {
            n956 = event-data() -> ()  [unwired: 1 in, 5 out]
            n957 = Number To Decimal String(number="Bias Voltage (mV)") -> (decimal integer string=w1510:string)  [unwired: 1 in]
            n958 = Number To Fractional String(number="Bias Voltage (mV)") -> (F-format string=w1505:string)  [unwired: 3 in]
            n959 = Concatenate Strings("BSLV " ("string"), w1510) -> (w1508:string)
            n960 = Concatenate Strings("bias voltage value ", w1505) -> (w1504:string)
          }
          event "Filter Type": Value Change {
            n961 = event-data() -> ()  [unwired: 1 in, 5 out]
            n962 = Concatenate Strings("FLTT " ("string"), "Filter Type") -> (w1511:string)
          }
          event "Lowpass 3dB Point": Value Change {
            n963 = event-data() -> ()  [unwired: 1 in, 5 out]
            n964 = Concatenate Strings("LFRQ " ("string"), "Lowpass 3dB Point") -> (w1515:string)
          }
          event "Highpass 3dB Point": Value Change {
            n965 = event-data() -> ()  [unwired: 1 in, 5 out]
            n966 = Concatenate Strings("HFRQ " ("string"), "Highpass 3dB Point") -> (w1518:string)
          }
          event "Filter Reset": Value Change {
            n967 = event-data() -> ()  [unwired: 1 in, 5 out]
            n968 = Select(t="ROLD", s="Filter Reset", f="") -> (s? t:f=w1521:string)
          }
          event "Gain Mode": Value Change {
            n969 = event-data() -> ()  [unwired: 1 in, 5 out]
            n970 = Concatenate Strings("GNMD " ("string"), "Gain Mode") -> (w1524:string)
          }
          event "Invert Signal": Value Change {
            n971 = event-data() -> ()  [unwired: 1 in, 5 out]
            n972 = Boolean To (0,1)(Boolean="Invert Signal") -> (0, 1=w1534:i16)
            n973 = Number To Decimal String(number=w1534) -> (decimal integer string=w1533:string)  [unwired: 1 in]
            n974 = Concatenate Strings("INVT " ("string"), w1533) -> (w1531:string)
            n975 = Select(t="signal inverted", s="Invert Signal", f="signal not inverted") -> (s? t:f=w1527:string)
          }
          event "Send Command": Value Change {
            n976 = event-data() -> ()  [unwired: 1 in, 5 out]
          }
        }
        "Command Sent" <- w1452
        n977 = local read "Save Event Log?"() -> (w1448:bool)
        n978 = local read "Saving..."() -> (w1449:bool)
        n979 = And(x=w1448, y=w1449) -> (x .and. y?=w1450:bool)
        n980 = case shown="True" w1450 {
          tunnel: w1447 -> [_ w1457]
          frame False {
          }
          frame True {
            n981 = local read "Time (s)"() -> (w1458:dbl)
            n982 = local read "log file ref"() -> (w1459:refnum<file>)
            n983 = call "write to event log.vi"("log file ref"=w1459, "time"=w1458, "input string"=w1457) -> ()  [unwired: 8 in]
          }
        }
        n984 = call "preamp serial write macro.vi"("String"=w1452, "Delay (ms)"=w1453, "VISA resource name"=w1456) -> ("read buffer"=→"Reply":string, "error out"=w1455:errorcluster)  [unwired: 1 out]
        n985 = call "preamp serial write macro.vi"("String"=w1452, "Delay (ms)"=w1453, "VISA resource name"=w1451) -> ()  [unwired: 3 out]
        n986 = local write "Preamp Error Out"(w1455) -> ()
      }
      event "Start slow trap scan": Value Change {
        n987 = event-data() -> ()  [unwired: 1 in, 5 out]
        n988 = while {
          tunnel: [FALSE] -> w1537
          tunnel: "Start slow trap scan" -> [_]
          i -> [w1553]
          stop <- w1541 stop-if-true
          # "number of steps"
          n989 = local read "Trap Delta (MHz)"() -> (w1543:dbl)
          n990 = Divide(x="Trap scan range (MHz) (slow scan)", y="Trap step increment (MHz) (slow scan)") -> (x/y=w1550:dbl)
          n991 = Wait (ms)(milliseconds to wait="Trap step dwell (ms) (slow scan)") -> ()  [unwired: 1 out]
          n992 = Sign(1:"Trap scan range (MHz) (slow scan)") -> (0:w1546:dbl)
          n993 = Multiply(x="Trap step increment (MHz) (slow scan)", y=w1546) -> (x*y=w1544:dbl)
          n994 = Add(x=w1544, y=w1543) -> (x+y=w1542:dbl)
          n995 = Absolute Value(x=w1550) -> (abs(x)=w1538:dbl)
          n996 = property on="Trap Delta (MHz)" class="DigNum (strict)"("Val(Sgnl)"=w1542) -> ()  [unwired: 2 in, 2 out]
          n997 = Increment(x=w1553) -> (x+1=w1539:i32)
          n998 = Greater Or Equal?(x=w1539, y=w1538) -> (x >= y?=w1552:bool)
          n999 = Or(x=w1552, y="Cancel slow trap scan") -> (x .or. y?=w1541:bool)
          "Scanning (slow scan)" <- TRUE ("Scanning (slow scan)")
        }
        n1000 = local write "Scanning (slow scan)"(w1537) -> ()
        n1001 = local write "Cancel slow trap scan"(w1537) -> ()
      }
      event "Start slow f-ext": Value Change {
        n1002 = event-data() -> ()  [unwired: 1 in, 5 out]
        n1003 = flat-sequence {
          tunnel: [w1560] -> w1556
          tunnel: w1556 -> [w1594]
          tunnel: [w1594] -> w1555
          tunnel: [w1608] -> w1557
          tunnel: w1555 -> [w1608]
          frame #0 {
            w1560 = FALSE ("Immediately quit scan")
            n1004 = case shown="True" "Read trap position file first" {
              frame False {
              }
              frame True {
                n1005 = local read "Save file name"() -> (w1566:path)
                n1006 = Strip Path(path=w1566) -> (stripped path=w1580:path)  [unwired: 1 out]
                n1007 = Path To String(path=w1580) -> (string=w1579:string)
                n1008 = Concatenate Strings(w1579, "\\trap_positions" ("string")) -> (w1577:string)
                n1009 = String To Path(string=w1577) -> (path=w1576:path)
                n1010 = Open/Create/Replace File(file path (use dialog)=w1576, operation (0:open)=T35."open", access (0:read/write)=enum16{"read/write", "read-only", "write-only"}."read-only") -> (refnum out=w1583:refnum<file>, error out=w1570:errorcluster)  [unwired: 1 in, 3 out]
                n1011 = Deny Access(4:w1570, 7:w1583) -> (0:w1569:errorcluster, 3:w1575:refnum<file>)  [unwired: 1 out]
                n1012 = Read from Binary File(5:0.0, 8:w1569, 9:T34."big-endian, network order" ("byte order (0:big-endian, network order)"), 10:-1 ("count (1)"), 11:w1575) -> (0:w1568:errorcluster, 2:w1561:dbl[], 3:w1571:refnum<file>)  [unwired: 2 out]
                n1013 = In Range and Coerce(upper limit=dbl[] [20.0, 20.0, 20.0] ("lower limit"), x=w1561, lower limit=dbl[] [10.0, 10.0, 10.0]) -> (In Range?=w1563:bool[])  [unwired: 1 out]
                n1014 = Close File(refnum=w1571, error in=w1568) -> (error out=→"Read trap position error":errorcluster)  [unwired: 1 out]
                n1015 = And Array Elements(Boolean array=w1563) -> (logical AND=w1562:bool)
                n1016 = case "Update if positions within range" shown="True" w1562 {
                  tunnel: w1561 -> [_ w1587]
                  frame False {
                    n1017 = local read "Messages"() -> (w1586:string)
                    n1018 = call <vilib>:"Beep.vi"() -> ()  [unwired: 12 in]
                    n1019 = call "Update messages.vi"("Message to add"="Trap positions outside allowed range.", "Old message string"=w1586) -> ("New message string"=w1585:string)
                    n1020 = local write "Messages"(w1585) -> ()
                  }
                  frame True {
                    n1021 = local write "Trap pause positions (MHz)"(w1587) -> ()
                  }
                }
              }
            }
            n1022 = local write "Immediately quit scan"(w1560) -> ()
            n1023 = local write "Cancel pause"(w1560) -> ()
            n1024 = local write "Pause scan"(w1560) -> ()
          }
          frame #1 {
            # "Quickly scan to starting position (jumping directly might lose beads)"
            n1025 = local read "Trap Delta (MHz)"() -> (w1591:dbl)
            n1026 = Index Array(array="Trap pause positions (MHz)", index=0) -> (element=w1588:dbl)
            n1027 = Subtract(x=w1588, y=w1591) -> (x-y=w1590:dbl)
            n1028 = Sign(1:w1590) -> (0:w1589:dbl)
            n1029 = while {
              tunnel: w1589 -> [w1606]
              tunnel: w1588 -> [w1598]
              stop <- w1596 stop-if-true
              # "0.1 MHz per step"
              # "50 ms per step"
              n1030 = local read "Trap Delta (MHz)"() -> (w1603:dbl)
              n1031 = Multiply(x=w1606, y=0.1) -> (x*y=w1604:dbl)
              n1032 = Add(x=w1604, y=w1603) -> (x+y=w1597:dbl)
              n1033 = Subtract(x=w1598, y=w1597) -> (x-y=w1602:dbl)
              n1034 = Absolute Value(x=w1602) -> (abs(x)=w1601:dbl)
              n1035 = Less?(x=w1601, y=0.3) -> (x < y?=w1596:bool)
              n1036 = Select(t=w1598, s=w1596, f=w1597) -> (s? t:f=w1599:dbl)
              n1037 = Wait (ms)(milliseconds to wait=u32 50) -> ()  [unwired: 1 out]
              n1038 = property on="Trap Delta (MHz)" class="DigNum (strict)"("Val(Sgnl)"=w1599) -> ()  [unwired: 2 in, 2 out]
            }
          }
          frame #2 {
            n1039 = case shown="True" "Start saving before pull" {
              frame False {
              }
              frame True {
                n1040 = property on="Start Saving" class="Bool (strict)"("Val(Sgnl)"=TRUE ("Value (Signaling)")) -> ()  [unwired: 2 in, 2 out]
              }
            }
          }
        }
        n1041 = while {
          tunnel: w1557 -> [_]
          tunnel: ["Stop saving when done"] -> w1554
          i -> [w1611]
          stop <- w1613 stop-if-true
          n1042 = flat-sequence {
            tunnel: [w1616] -> w1614
            tunnel: w1611 -> [w1615]
            tunnel: w1614 -> [w1666]
            tunnel: [w1725] -> w1613
            tunnel: w1611 -> [w1729]
            frame #0 {
              # "Pull"
              n1043 = while {
                shift-right: [w1640] -> _
                shift-left: TRUE -> [w1639]
                tunnel: ["Stop pulling and reverse"] -> w1616
                tunnel: w1615 -> [w1623]
                stop <- w1645 stop-if-true
                n1044 = local read "Trap pause positions (MHz)"() -> (w1627:dbl[])
                n1045 = local read "Trap Delta (MHz)"() -> (w1632:dbl)
                n1046 = Wait (ms)(milliseconds to wait="Trap step dwell (ms) (slow scan) 2") -> ()  [unwired: 1 out]
                n1047 = local write "Cancel pause"(FALSE ("Cancel pause")) -> ()
                n1048 = Select(t=0.0, s="Pause scan", f="Trap step increment (MHz) (slow scan) 2") -> (s? t:f=w1636:dbl)
                n1049 = Index Array(array=w1627, index=2) -> (element=w1629:dbl)
